vi "Read Element by Index.vi"(8 "error in (no error)":errorcluster, 10 "index":i32, 11 "MusicElementLibrary in":refnum<class "MusicElementLibrary.lvclass">) -> (0 "error out":errorcluster, 2 "MusicElement.lvclass":refnum<class "MusicElement.lvclass">, 3 "MusicElementLibrary out":refnum<class "MusicElementLibrary.lvclass">, 5 "Found?":bool)   [LabVIEW 2015, in "MusicElementLibrary.lvclass"]
uses:
  MusicElementLibrary.lvclass
  MusicElement.lvclass
  MusicElementLibrary.lvclass/MusicElementLibrary.ctl
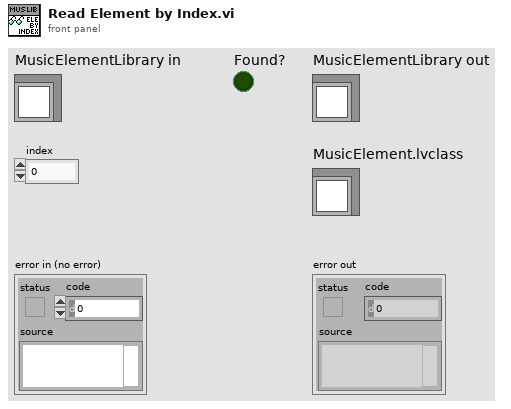
[diagram p1: front panel]
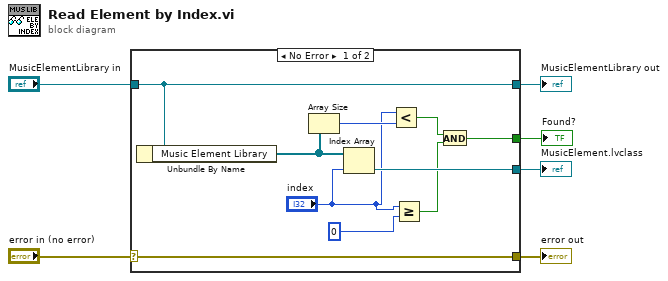
[diagram p0: block diagram]
diagram:
  n1 = case shown="No Error" "error in (no error)" {
    selector: "error in (no error)" -> [w16 w17]
    tunnel: [w16 w17] -> w5
    tunnel: [w15 w18] -> w3
    tunnel: "MusicElementLibrary in" -> [w15 w18]
    tunnel: [w14 _] -> w2
    tunnel: [w10 _] -> w1
    frame No Error {
      n2 = Unbundle By Name(w15) -> ("Music Element Library"=w13:refnum<class "MusicElement.lvclass">[])
      n3 = Array Size(array=w13) -> (size(s)=w12:i32)
      n4 = Index Array(array=w13, index="index") -> (element=w14:refnum<class "MusicElement.lvclass">)
      n5 = Less?(x="index", y=w12) -> (x < y?=w11:bool)
      n6 = Greater Or Equal?(x="index", y=0 ("lower limit")) -> (x >= y?=w7:bool)
      n7 = And(x=w11, y=w7) -> (x .and. y?=w10:bool)
    }
    frame Error {
    }
  }
  "error out" <- w5
  "MusicElementLibrary out" <- w3
  "MusicElement.lvclass" <- w2
  "Found?" <- w1
